vi "Periodic Tasks.vi"(8 "error in":errorcluster) -> ()   [LabVIEW 2016]
doc: "This VI runs in parallel to other tasks. It can contain as many user-defined periodic loops as you need. These can carry out PID or other sorts of timed response."
uses:
  Robot Global Data.vi
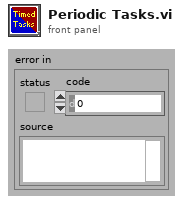
[diagram p1: front panel]
types:
  T1 = typedef "WPI_EncoderDevRef.ctl" = cluster{"DevStatus":errorcluster, "EncoderIndex":T2, "CounterIndex":T3, "DistancePerCount":dbl, "Decoding Type":T4}
  T2 = typedef "FPGA_EncoderIdx.ctl" = enum8{"Enc 0", "Enc 1", "Enc 2", "Enc 3", "Enc 4", "Enc 5", "Enc 6", "Enc 7", "Invalid"}
  T3 = typedef "FPGA_CounterCtrSystemIndex.ctl" = enum8{"Ctr 0", "Ctr 1", "Ctr 2", "Ctr 3", "Ctr 4", "Ctr 5", "Ctr 6", "Ctr 7", "Invalid"}
  T4 = typedef "WPI_EncoderType.ctl" = enum16{"1x", "2x", "4x"}
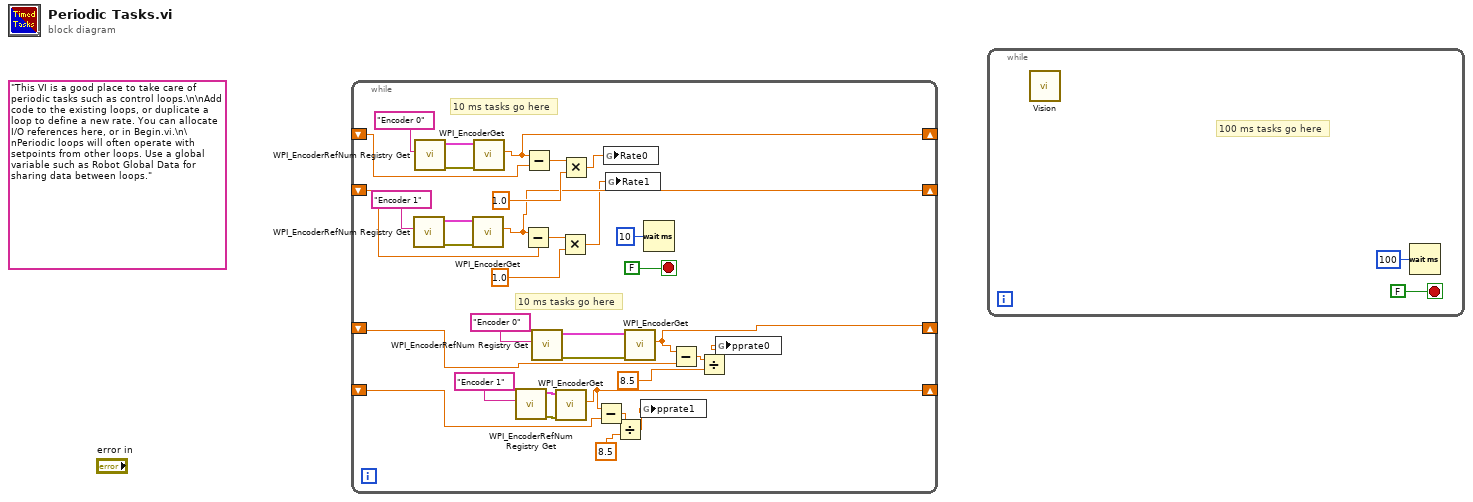
[diagram p0: block diagram]
diagram:
  (unwired) "This VI is a good place to take care of periodic tasks such as control loops.\n\nAdd code to the existing loops, or duplicate a loop to define a new rate. You can allocate I/O references here, or in Begin.vi.\n\nPeriodic loops will often operate with setpoints from other loops. Use a global variable such as Robot Global Data for sharing data between loops."
  n1 = while {
    shift-right: [w29] -> _
    shift-left: _ -> [w28]
    shift-right: [w19] -> _
    shift-left: _ -> [w20]
    shift-right: [w4] -> _
    shift-left: _ -> [w3]
    shift-right: [w2] -> _
    shift-left: _ -> [w1]
    stop <- FALSE stop-if-true
    # "10 ms tasks go here"
    # "10 ms tasks go here"
    n2 = call <vilib>:"WPI_EncoderRefNum Registry Get.vi"("refnum name"="Encoder 1") -> ("error out"=w25:errorcluster, "EncoderDevRef"=w24:T1)  [unwired: 9 in]
    n3 = call <vilib>:"WPI_EncoderRefNum Registry Get.vi"("refnum name"="Encoder 0") -> ("error out"=w32:errorcluster, "EncoderDevRef"=w31:T1)  [unwired: 9 in]
    n4 = call <vilib>:"WPI_EncoderGet.vi"("error in (no error)"=w25, "EncoderDevRef"=w24) -> ("Distance"=w19:dbl)  [unwired: 4 in, 5 out]
    n5 = call <vilib>:"WPI_EncoderGet.vi"("error in (no error)"=w32, "EncoderDevRef"=w31) -> ("Distance"=w29:dbl)  [unwired: 4 in, 5 out]
    n6 = call <vilib>:"WPI_EncoderRefNum Registry Get.vi"("refnum name"="Encoder 1") -> ("error out"=w11:errorcluster, "EncoderDevRef"=w12:T1)  [unwired: 9 in]
    n7 = Subtract(x=w19, y=w20) -> (x-y=w23:dbl)
    n8 = Subtract(x=w29, y=w28) -> (x-y=w27:dbl)
    n9 = call <vilib>:"WPI_EncoderRefNum Registry Get.vi"("refnum name"="Encoder 0") -> ("error out"=w13:errorcluster, "EncoderDevRef"=w14:T1)  [unwired: 9 in]
    n10 = call <vilib>:"WPI_EncoderGet.vi"("error in (no error)"=w11, "EncoderDevRef"=w12) -> ("Distance"=w2:dbl)  [unwired: 4 in, 5 out]
    n11 = Multiply(x=w23, y=1.0) -> (x*y=w17:dbl)
    n12 = Multiply(x=w27, y=1.0) -> (x*y=w18:dbl)
    n13 = Subtract(x=w2, y=w1) -> (x-y=w10:dbl)
    n14 = global write "Robot Global Data.vi" "Rate0"(w18) -> ()
    n15 = global write "Robot Global Data.vi" "Rate1"(w17) -> ()
    n16 = Divide(x=w10, y=8.5) -> (x/y=w9:dbl)
    n17 = call <vilib>:"WPI_EncoderGet.vi"("error in (no error)"=w13, "EncoderDevRef"=w14) -> ("Distance"=w4:dbl)  [unwired: 4 in, 5 out]
    n18 = global write "Robot Global Data.vi" "pprate1"(w9) -> ()
    n19 = Wait (ms)(milliseconds to wait=u32 10) -> ()  [unwired: 1 out]
    n20 = Subtract(x=w4, y=w3) -> (x-y=w6:dbl)
    n21 = Divide(x=w6, y=8.5) -> (x/y=w8:dbl)
    n22 = global write "Robot Global Data.vi" "pprate0"(w8) -> ()
  }
  n23 = while {
    stop <- FALSE stop-if-true
    # "100 ms tasks go here"
    n24 = call "Vision.vi"() -> ()  [unwired: 12 in]
    n25 = Wait (ms)(milliseconds to wait=u32 100) -> ()  [unwired: 1 out]
  }
